vi "get swerve drive pos.vi"(8 "error in (no error)":errorcluster) -> (0 "error out":errorcluster, 2 "Get POS":dbl[](array[numeric]))   [LabVIEW 2023]
uses:
  Global INIT.vi
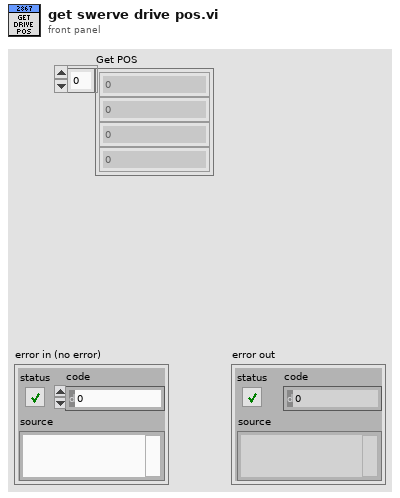
[diagram p1: front panel]
types:
  T1 = typedef "ctrl swerve motor.ctl" = cluster{"description":string, "MOTOR SELECT":T2, "Installed?":bool, "CAN ID":u8, "refnum name":string, "Invert":bool, "Idle Mode":T3, "Current limiting":T4, "MOTOR PIDF coefficients":T5, "gear ratio":dbl}
  T2 = typedef "ctrl MOTOR SELECT.ctl" = i16
  T3 = typedef "Spark MAX Idle Mode.ctl" = enum16{"Coast", "Brake"}
  T4 = typedef "ctrl Spark MAX current limiting.ctl" = cluster{"Linearized":bool, "Free Speed (A)":dbl, "Primay (A)":dbl, "Limit RPM (0)":u32}
  T5 = typedef "ctrl motor PIDF coefficients.ctl" = cluster{"PIDF":cluster{"P Gain":dbl, "I Gain":dbl, "D Gain":dbl, "F Gain":dbl, "I Zone":dbl, "Min Output":dbl, "Max Output":dbl}, "Smart Motion":T6}
  T6 = typedef "Spark MAX Smart Motion Parameters.ctl" = cluster{"Max Velocity":dbl, "Max Acceleration":dbl, "Minimum Velocity Output":dbl, "Allowed Closed Loop Error":dbl}
  T7 = typedef "WPI_MotorControlDeviceRef.ctl" = cluster{"DeviceStatus":errorcluster, "Type":T8, "PWM":cluster{"PWM Channel":T9, "DeadBand":T10}, "CAN":cluster{"Device Number":u8, "SetOutput VI Ref":variant, "GetOutput VI Ref":variant, "Enable VI Ref":variant, "Disable VI Ref":variant, "Data":variant}, "Invert":bool, "DIO PWM":cluster{"PWM \"Enable\" Channel":T9, "DIOChannel":T11, "PWM Rate":dbl}}
  T8 = typedef "WPI_MotorControlType.ctl" = enum16{"PWM", "CAN", "DIO PWM"}
  T9 = typedef "FPGA_DIOPWMChannel.ctl" = enum8{"PWM 0", "PWM 1", "PWM 2", "PWM 3", "PWM 4", "PWM 5", "PWM 6", "PWM 7", "PWM 8", "PWM 9", "PWM MXP 0", "PWM MXP 1", "PWM MXP 2", "PWM MXP 3", "PWM MXP 4", "PWM MXP 5", "PWM MXP 6", "PWM MXP 7", "PWM MXP 8", "PWM MXP 9", "Invalid"}
  T10 = typedef "WPI_PWMDeadband.ctl" = cluster{"Name":string, "maxPositivePwm":i32, "minPositivePwm":i32, "centerPwm":i32, "maxNegativePwm":i32, "minNegativePwm":i32, "angularRange":u16}
  T11 = typedef "FPGA_DIOChannel.ctl" = enum8{"DIO 0", "DIO 1", "DIO 2", "DIO 3", "DIO 4", "DIO 5", "DIO 6", "DIO 7", "DIO 8", "DIO 9", "DIO MXP 0", "DIO MXP 1", "DIO MXP 2", "DIO MXP 3", "DIO MXP 4", "DIO MXP 5", "DIO MXP 6", "DIO MXP 7", "DIO MXP 8", "DIO MXP 9", "DIO MXP 10", "DIO MXP 11", "DIO MXP 12", "DIO MXP 13", "DIO MXP 14", "DIO MXP 15", "SPI Port CS1", "SPI Port CS2", "SPI Port CS3", "SPI Port MISO", "SPI Port MOSI", "Invalid"}
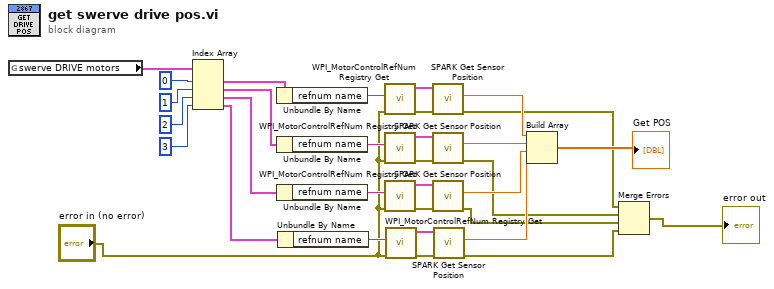
[diagram p0: block diagram]
diagram:
  n1 = global read "Global INIT.vi" "swerve DRIVE motors"() -> (w29:T1[])
  n2 = Index Array(array=w29, index #1=0 ("index"), index #2=1 ("index"), index #3=2 ("index"), index #4=3 ("index")) -> (element #1=w19:T1, element #2=w18:T1, element #3=w17:T1, element #4=w16:T1)
  n3 = Unbundle By Name(w19) -> ("refnum name"=w32:string)
  n4 = Unbundle By Name(w18) -> ("refnum name"=w28:string)
  n5 = Unbundle By Name(w17) -> ("refnum name"=w25:string)
  n6 = Unbundle By Name(w16) -> ("refnum name"=w22:string)
  n7 = call <vilib>:"WPI_MotorControlRefNum Registry Get.vi"("error in (no error)"="error in (no error)", "refnum name"=w32) -> ("error out"=w31:errorcluster, "MotorControlDevRef"=w30:T7)  [unwired: 8 in]
  n8 = call <vilib>:"WPI_MotorControlRefNum Registry Get.vi"("error in (no error)"="error in (no error)", "refnum name"=w28) -> ("error out"=w27:errorcluster, "MotorControlDevRef"=w26:T7)  [unwired: 8 in]
  n9 = call <vilib>:"WPI_MotorControlRefNum Registry Get.vi"("error in (no error)"="error in (no error)", "refnum name"=w25) -> ("error out"=w24:errorcluster, "MotorControlDevRef"=w23:T7)  [unwired: 8 in]
  n10 = call <vilib>:"WPI_MotorControlRefNum Registry Get.vi"("error in (no error)"="error in (no error)", "refnum name"=w22) -> ("error out"=w21:errorcluster, "MotorControlDevRef"=w20:T7)  [unwired: 8 in]
  n11 = call <vilib>:"SPARK Get Sensor Position.vi"("error in (no error)"=w31, "MotorControlDevRef in"=w30) -> ("error out"=w6:errorcluster, "Sensor Position"=w11:dbl)  [unwired: 6 in, 2 out]
  n12 = call <vilib>:"SPARK Get Sensor Position.vi"("error in (no error)"=w27, "MotorControlDevRef in"=w26) -> ("error out"=w5:errorcluster, "Sensor Position"=w10:dbl)  [unwired: 6 in, 2 out]
  n13 = call <vilib>:"SPARK Get Sensor Position.vi"("error in (no error)"=w24, "MotorControlDevRef in"=w23) -> ("error out"=w4:errorcluster, "Sensor Position"=w9:dbl)  [unwired: 6 in, 2 out]
  n14 = call <vilib>:"SPARK Get Sensor Position.vi"("error in (no error)"=w21, "MotorControlDevRef in"=w20) -> ("error out"=w3:errorcluster, "Sensor Position"=w8:dbl)  [unwired: 6 in, 2 out]
  n15 = Build Array(w11, w10, w9, w8) -> (→"Get POS":dbl[])
  n16 = Merge Errors(w6, w5, w4, w3) -> (→"error out":errorcluster)
